vi "Test_memory_scope.vi"() -> ()   [LabVIEW 2013]
uses:
  <vilib>/userdefined/High Color/nirio_resource_hc.ctl
  Scope5782/Scope/controls/scope_params_5782.ctl
  Utilities/Ticker/Ticker.lvclass
  Communication/Driver/RemoteConnection/RemoteConnection.lvclass
  Scope/controls/ScopeMode.ctl
  Scope5782/Config/FPGAref_5782.ctl
  FPGA/DataMode.ctl
  Scope5782/Scope/controls/5782_trigger_type.ctl
  Scope5782/Scope/controls/Feedforward.ctl
  Scope5782/Scope/controls/Memory block.ctl
  <vilib>/FPGAPlugInAG/PXIe-7975R/niLvFpga_Open_PXIe-7975R.vi
  <vilib>/rvi/interface/common/dynamic/niFpgaDynamicAddResources.vi
  <vilib>/rvi/interface/common/niFpgaWaitOnOcc.vi
  <vilib>/Utility/error.llb/Error Cluster From Error Code.vi
  <vilib>/rvi/errors/niLvFpgaAdjustHostInterfaceError.vi
  <vilib>/FPGAPlugInAG/Dynamic/niLvFpga_Close_Dynamic.vi
  <vilib>/rvi/interface/nirviOpenFPGA/nirviOpenFPGA.xnode
  FPGA Bitfiles/Test_feed_forward1_OTIf-jJYddg.lvbitx
  <vilib>/rvi/interface/nirviMethod/nirviMethod.xnode
  <vilib>/rvi/interface/nirviReadWriteControl/nirviReadWriteControl.xnode
  <vilib>/rvi/interface/nirviCloseFPGA/nirviCloseFPGA.xnode
  <vilib>/rvi/interface/Simulation/niFpgaSimulationCallBeginRW.vi
  <vilib>/FPGAPlugInAG/Dynamic/niLvFpga_ReadFifo_Dynamic.vi
  <vilib>/rvi/errors/niLvFpgaMergeErrorWithErrorCode.vi
  <vilib>/FPGAPlugInAG/Dynamic/niLvFpga_ConfigureFifo_Dynamic.vi
  <vilib>/FPGAPlugInAG/Dynamic/niLvFpga_StartFifo_Dynamic.vi
  NiFpgaLv.dll
panel:
  out "Actual Depth 2":u32
  out "Actual Depth":u32
  in  "fetch":bool
  in  "stop":bool
  in  "scope in":T1
  in  "Beam/FF enabled":bool
  in  "show beam":bool
  in  "Beam":path
  out "error out":errorcluster
  out "Waveform Graph":dbl[][](graph)
  out "Configured?":bool
  out "Clocking Option Configured?":bool
  in  "resource name":T7="PXI1Slot18"
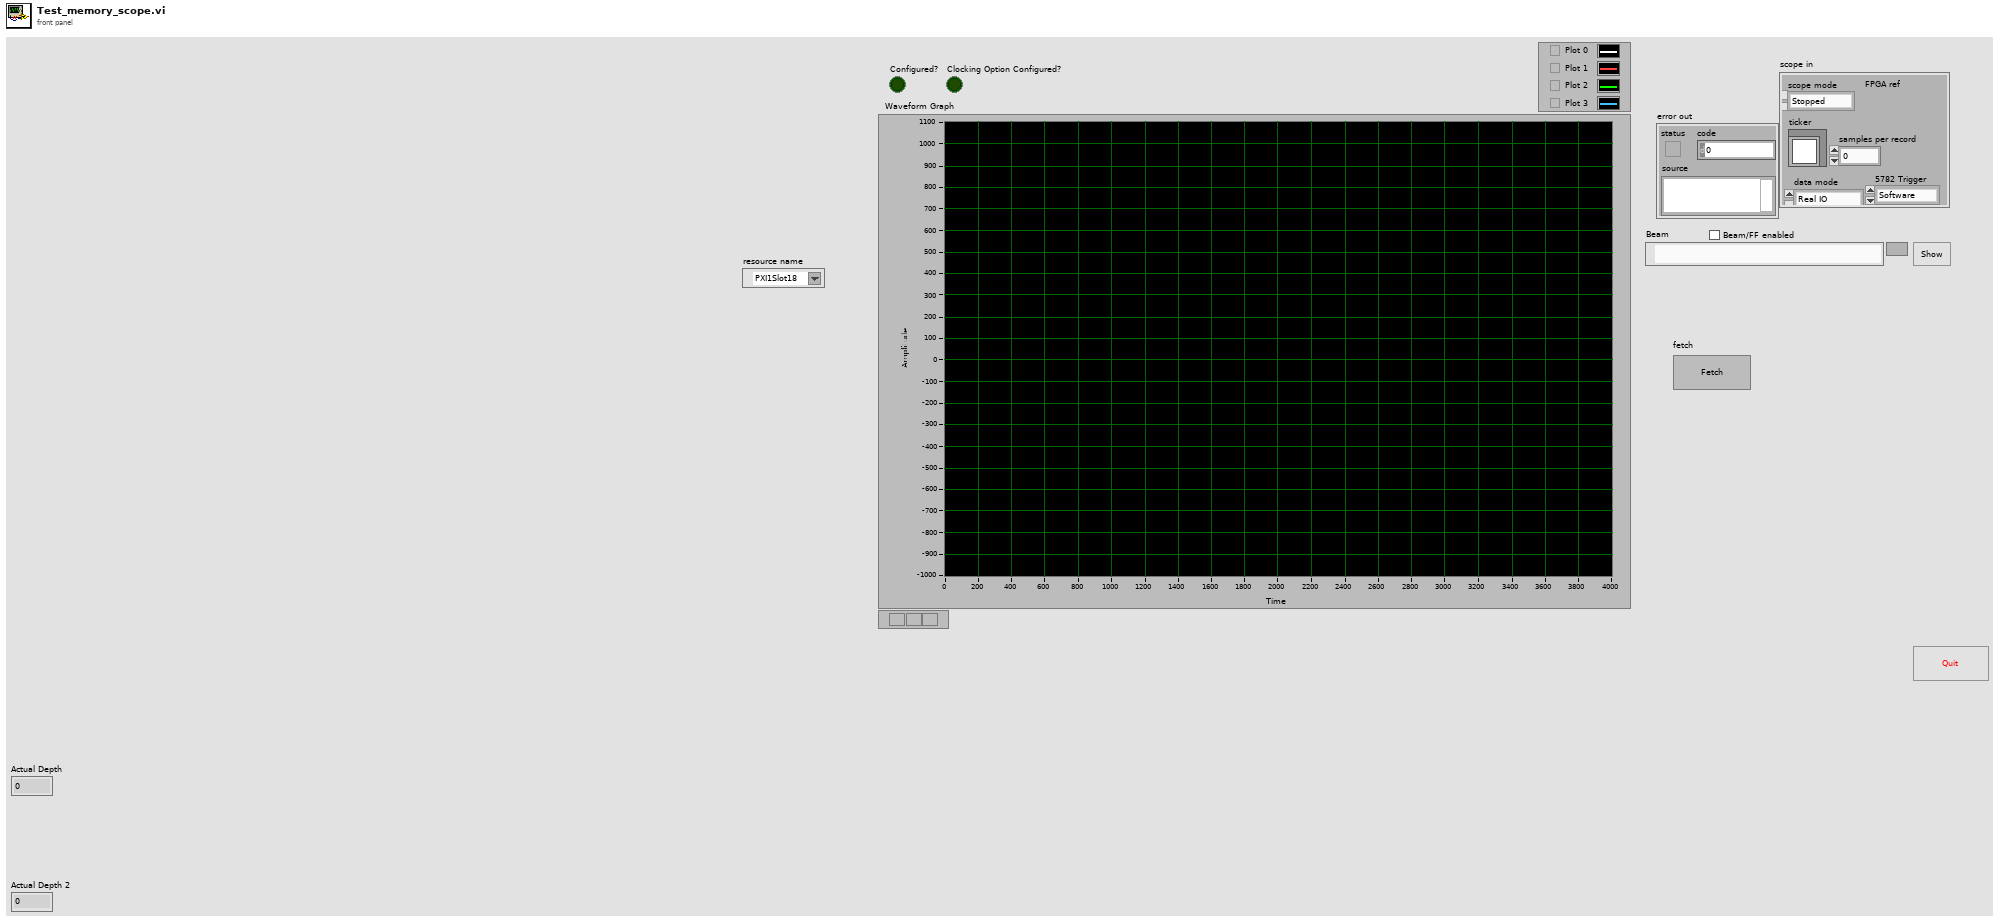
[diagram p1: front panel]
types:
  T1 = typedef "scope_params_5782.ctl" = cluster{"scope mode":T2, "ticker":refnum<class "Ticker.lvclass">, "samples per record":i32, "FPGA ref":T3, "data mode":T4, "5782 Trigger":T5, "Chart length":i32, "RemoteConnection":refnum<class "RemoteConnection.lvclass">, "last phase":dbl[], "Feedforward":T6}
  T2 = typedef "ScopeMode.ctl" = enum16{"Stopped", "Single", "Running", "Continuous"}
  T3 = typedef "FPGAref_5782.ctl" = refnum<k20>
  T4 = typedef "DataMode.ctl" = enum16{"Real IO", "Simulated"}
  T5 = typedef "5782_trigger_type.ctl" = enum16{"Software", "Trigger input"}
  T6 = typedef "Feedforward.ctl" = cluster{"Beam I":dbl[], "Beam Q":dbl[], "Feedforward I":dbl[], "Feedforward Q":dbl[], "Setpoint I":dbl[], "Setpoint Q":dbl[]}
  T7 = typedef "nirio_resource_hc.ctl" = tag
  T8 = enum8{"Internal Clock PLL Off", "Internal Clock PLL On (REF IN)", "External Clock (CLK_IN)", "Internal Clock PLL On (IoModSyncClk)"}
  T9 = typedef "Memory block.ctl" = enum16{"Setpoint", "Beam"}
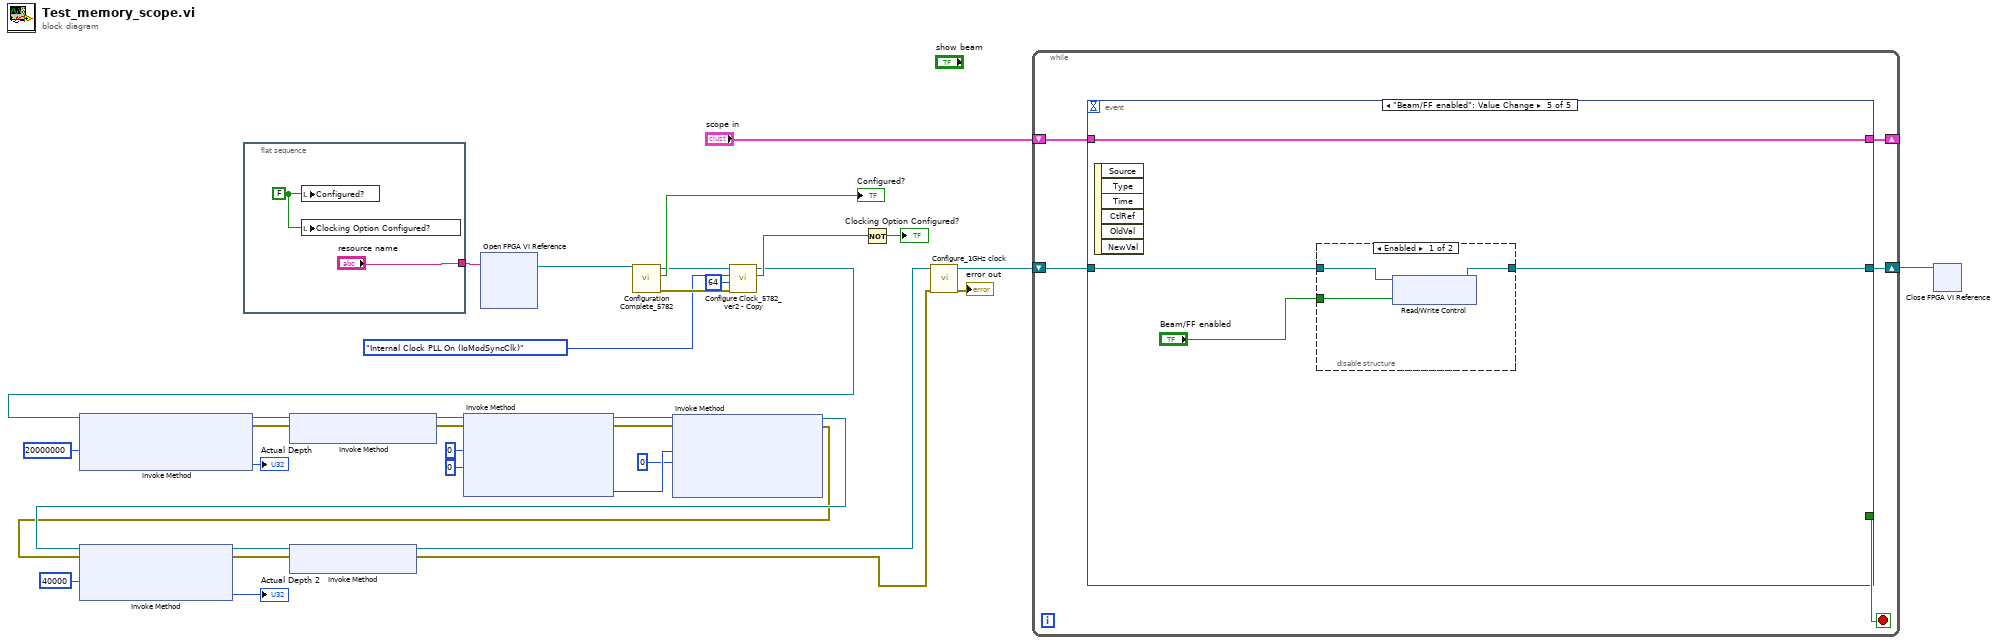
[diagram p0: block diagram]
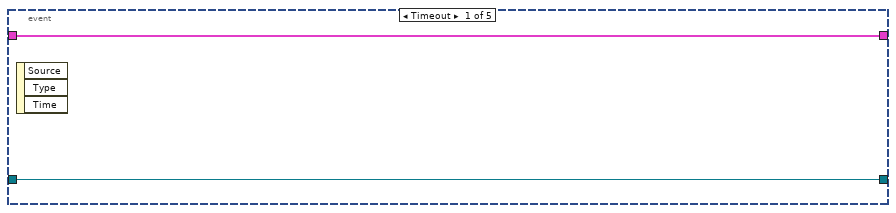
[diagram p2: hidden frame]
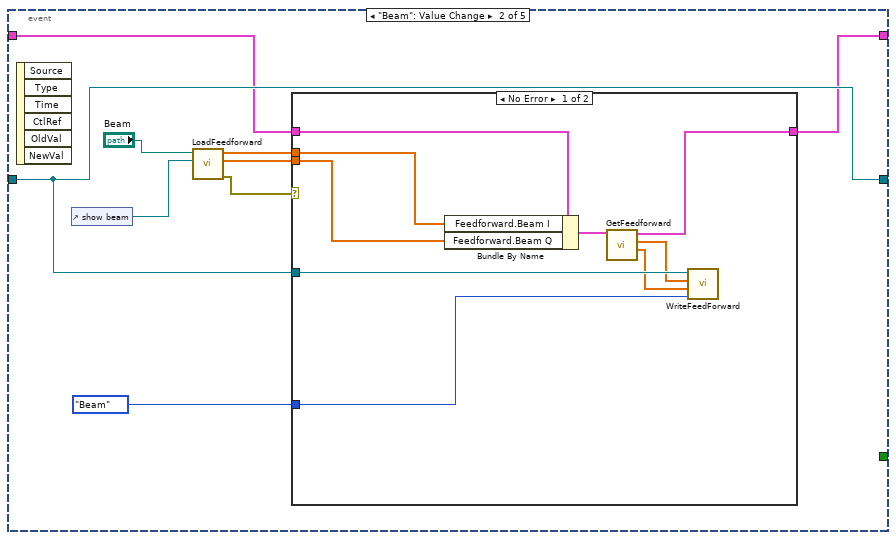
[diagram p3: hidden frame]
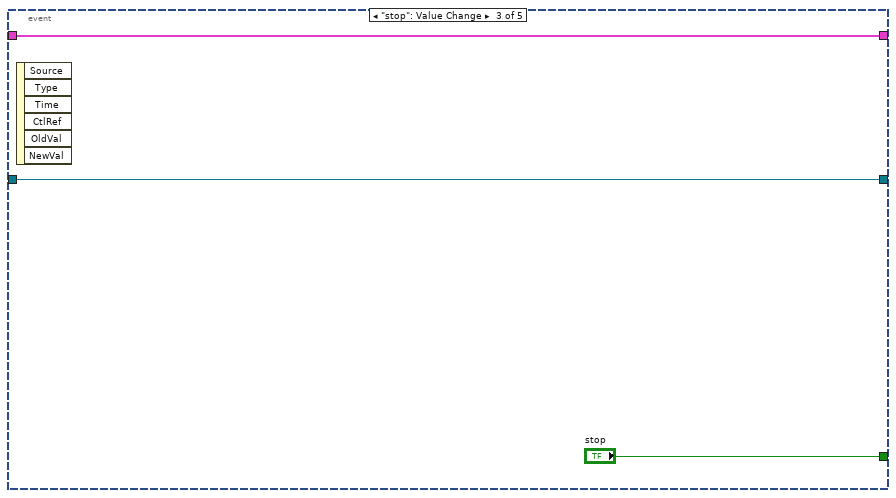
[diagram p5: hidden frame]
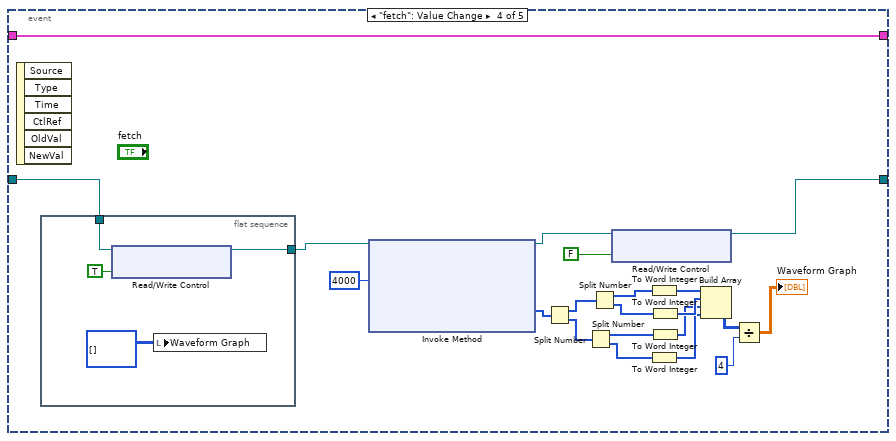
[diagram p6: hidden frame]
diagram:
  n1 = flat-sequence {
    tunnel: ["resource name"] -> w31
    frame #0 {
      w35 = FALSE ("Configured?")
      n2 = local write "Configured?"(w35) -> ()
      n3 = local write "Clocking Option Configured?"(w35) -> ()
    }
  }
  n4 = xnode "Open FPGA VI Reference"("resource name"=w31) -> ("FPGA VI Reference Out"=w23:refnum<k20>)  [unwired: 1 in, 1 out]
  n5 = call "Configuration Complete_5782.vi"("FPGA VI Reference in"=w23) -> ("error out"=w33:errorcluster, "Configured?"=→"Configured?":bool, "FPGA VI Reference out"=w22:refnum<k20>)  [unwired: 8 in]
  n6 = call "Configure Clock_5782_ver2 - Copy.vi"("error in"=w33, "User Data 1"=u8 64, "Clock Source"=T8."Internal Clock PLL On (IoModSyncClk)", "FPGA VI Reference"=w22) -> ("Configuration Error"=w29:bool, "FPGA VI Reference out"=w9:refnum<k20>)  [unwired: 5 in, 1 out]
  n7 = xnode "Invoke Method"("FPGA VI Reference In"=w9, "Requested Depth"=u32 20000000 ("Depth")) -> ("FPGA VI Reference Out"=w19:refnum<k20>, "error out"=w20:errorcluster, "Actual Depth"=→"Actual Depth":u32)  [unwired: 1 in]
  n8 = xnode "Invoke Method"("FPGA VI Reference In"=w19, "error in"=w20) -> ("FPGA VI Reference Out"=w11:refnum<k20>, "error out"=w10:errorcluster)
  n9 = xnode "Invoke Method"("FPGA VI Reference In"=w11, "error in"=w10, "Number of Elements"=u32 0, "Timeout (ms)"=0) -> ("FPGA VI Reference Out"=w14:refnum<k20>, "error out"=w13:errorcluster, "Elements Remaining"=w16:u32)  [unwired: 1 out]
  n10 = xnode "Invoke Method"("FPGA VI Reference In"=w14, "error in"=w13, "Number of Elements"=w16, "Timeout (ms)"=0) -> ("FPGA VI Reference Out"=w4:refnum<k20>, "error out"=w1:errorcluster)  [unwired: 2 out]
  n11 = xnode "Invoke Method"("FPGA VI Reference In"=w4, "error in"=w1, "Requested Depth"=u32 40000 ("Depth")) -> ("FPGA VI Reference Out"=w7:refnum<k20>, "error out"=w6:errorcluster, "Actual Depth"=→"Actual Depth 2":u32)
  n12 = xnode "Invoke Method"("FPGA VI Reference In"=w7, "error in"=w6) -> ("FPGA VI Reference Out"=w3:refnum<k20>, "error out"=w2:errorcluster)
  n13 = Not(x=w29) -> (.not. x?=→"Clocking Option Configured?":bool)
  n14 = call "Configure_1GHz clock.vi"("error in"=w2, "FPGA SPI config ref"=w3) -> ("error out"=→"error out":errorcluster, "FPGA SPI config out"=w27:refnum<k20>)  [unwired: 8 in]
  n15 = while {
    shift-right: [w38] -> w24
    shift-left: w27 -> [w41]
    shift-right: [w39] -> _
    shift-left: "scope in" -> [w40]
    stop <- w37 stop-if-true
    n16 = event shown="[4] \"Beam/FF enabled\": Value Change" {
      selector: _ -> [_ _ _ _ _]
      dyn-events: _ -> [_ _ _ _ _]
      timeout: _ -> [_ _ _ _ _]
      tunnel: w41 -> [w42 w47 w64 w85 w93]
      tunnel: w40 -> [w43 w45 w65 w86 w94]
      tunnel: [w43 w44 w65 w86 w94] -> w39
      tunnel: [w42 w47 w64 w69 w92] -> w38
      tunnel: [_ _ "stop" _ _] -> w37
      event Timeout {
        n17 = event-data() -> ()  [unwired: 1 in, 3 out]
      }
      event "Beam": Value Change {
        n18 = event-data() -> ()  [unwired: 1 in, 6 out]
        n19 = control-ref of="show beam"() -> (w48:refnum<vi>)
        n20 = call "LoadFeedforward.vi"("show ref"=w48, "Path"="Beam") -> ("error out"=w50:errorcluster, "values Q"=w52:dbl[], "values I"=w51:dbl[])  [unwired: 7 in]
        n21 = case shown="No Error" w50 {
          tunnel: w45 -> [w59 w62]
          tunnel: w52 -> [w60 _]
          tunnel: w51 -> [w61 _]
          tunnel: [w53 w62] -> w44
          tunnel: w47 -> [w57 _]
          tunnel: Memory_block."Beam" ("Memory block") -> [w58 _]
          frame No Error {
            n22 = Bundle By Name(cluster=w59, "Feedforward.Beam I"=w61, "Feedforward.Beam Q"=w60) -> (w56:T1)
            n23 = call "GetFeedforward.vi"("scope in"=w56) -> ("values Q"=w54:dbl[], "values I"=w55:dbl[], "scope out"=w53:T1)  [unwired: 8 in]
            n24 = call "WriteFeedForward.vi"("Memory block"=w58, "values Q"=w54, "values I"=w55, "FPGA VI Reference"=w57) -> ()  [unwired: 7 in, 1 out]
          }
          frame Error {
          }
        }
      }
      event "stop": Value Change {
        n25 = event-data() -> ()  [unwired: 1 in, 6 out]
      }
      event "fetch": Value Change {
        n26 = event-data() -> ()  [unwired: 1 in, 6 out]
        n27 = flat-sequence {
          tunnel: w85 -> [w90]
          tunnel: [w88] -> w84
          frame #0 {
            n28 = xnode "Read/Write Control"("FPGA VI Reference In"=w90, "Trigger Acquisition"=TRUE) -> ("FPGA VI Reference Out"=w88:refnum<k20>)  [unwired: 1 in, 1 out]
            n29 = local write "Waveform Graph"(i16[][] [] ("Waveform Graph")) -> ()
          }
        }
        n30 = xnode "Invoke Method"("FPGA VI Reference In"=w84, "Number of Elements"=u32 4000) -> ("FPGA VI Reference Out"=w71:refnum<k20>, "Data"=w76:u64[])  [unwired: 2 in, 2 out]
        n31 = Split Number(x=w76) -> (hi(x)=w81:u32[], lo(x)=w77:u32[])
        n32 = Split Number(x=w77) -> (hi(x)=w79:u16[], lo(x)=w80:u16[])
        n33 = Split Number(x=w81) -> (hi(x)=w82:u16[], lo(x)=w78:u16[])
        n34 = xnode "Read/Write Control"("FPGA VI Reference In"=w71, "Trigger Acquisition"=FALSE) -> ("FPGA VI Reference Out"=w69:refnum<k20>)  [unwired: 1 in, 1 out]
        n35 = To Word Integer(number=w82) -> (16bit integer=w75:i16[])
        n36 = To Word Integer(number=w80) -> (16bit integer=w72:i16[])
        n37 = To Word Integer(number=w78) -> (16bit integer=w74:i16[])
        n38 = To Word Integer(number=w79) -> (16bit integer=w73:i16[])
        n39 = Build Array(w75, w74, w73, w72) -> (w68:i16[][])
        n40 = Divide(x=w68, y=4) -> (x/y=→"Waveform Graph":dbl[][])
      }
      event "Beam/FF enabled": Value Change {
        n41 = event-data() -> ()  [unwired: 1 in, 6 out]
        n42 = disable-structure shown="Enabled" {
          disable-tunnel: w93 -> [w97 w98]
          disable-tunnel: [w96 w98] -> w92
          disable-tunnel: "Beam/FF enabled" -> [w95 _]
          frame Enabled {
            n43 = xnode "Read/Write Control"("FPGA VI Reference In"=w97, "Beam enabled"=w95) -> ("FPGA VI Reference Out"=w96:refnum<k20>)  [unwired: 1 in, 1 out]
          }
          frame Disabled {
          }
        }
      }
    }
  }
  n44 = xnode "Close FPGA VI Reference"("FPGA VI Reference In"=w24) -> ()  [unwired: 1 in, 1 out]
